vi "FTW-TestBootstrapper.vi"   [LabVIEW 2015, in "FTW-TestBootstrapper.lvclass"]
uses:
  FTW-TestBootstrapper.lvclass
panel:
  # "Static links to all FTW tests"
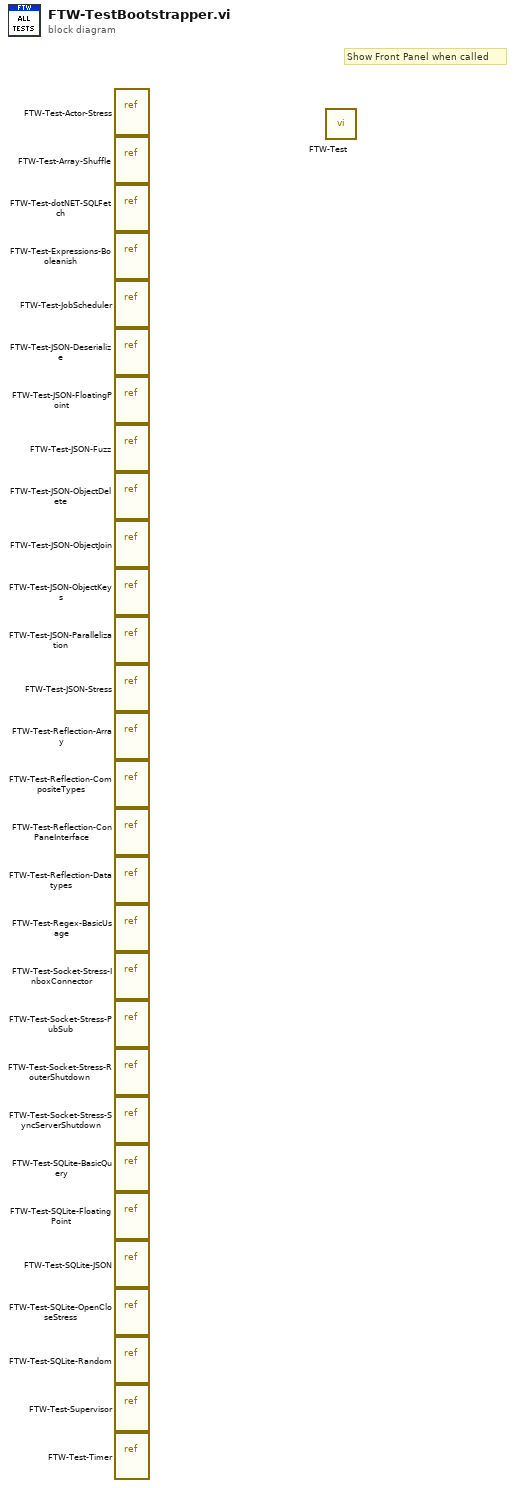
[diagram p0: block diagram]
diagram:
  # "Show Front Panel when called"
  n1 = vi-ref "FTW-Test-Actor-Stress.vi"() -> ()  [unwired: 1 out]
  n2 = vi-ref "FTW-Test-Array-Shuffle.vi"() -> ()  [unwired: 1 out]
  n3 = vi-ref "FTW-Test-dotNET-SQLFetch.vi"() -> ()  [unwired: 1 out]
  n4 = vi-ref "FTW-Test-Expressions-Booleanish.vi"() -> ()  [unwired: 1 out]
  n5 = vi-ref "FTW-Test-JobScheduler.vi"() -> ()  [unwired: 1 out]
  n6 = vi-ref "FTW-Test-JSON-Deserialize.vi"() -> ()  [unwired: 1 out]
  n7 = vi-ref "FTW-Test-JSON-FloatingPoint.vi"() -> ()  [unwired: 1 out]
  n8 = vi-ref "FTW-Test-JSON-Fuzz.vi"() -> ()  [unwired: 1 out]
  n9 = vi-ref "FTW-Test-JSON-ObjectDelete.vi"() -> ()  [unwired: 1 out]
  n10 = vi-ref "FTW-Test-JSON-ObjectJoin.vi"() -> ()  [unwired: 1 out]
  n11 = vi-ref "FTW-Test-JSON-ObjectKeys.vi"() -> ()  [unwired: 1 out]
  n12 = vi-ref "FTW-Test-JSON-Parallelization.vi"() -> ()  [unwired: 1 out]
  n13 = vi-ref "FTW-Test-JSON-Stress.vi"() -> ()  [unwired: 1 out]
  n14 = vi-ref "FTW-Test-Reflection-Array.vi"() -> ()  [unwired: 1 out]
  n15 = vi-ref "FTW-Test-Reflection-CompositeTypes.vi"() -> ()  [unwired: 1 out]
  n16 = vi-ref "FTW-Test-Reflection-ConPaneInterface.vi"() -> ()  [unwired: 1 out]
  n17 = vi-ref "FTW-Test-Reflection-Datatypes.vi"() -> ()  [unwired: 1 out]
  n18 = vi-ref "FTW-Test-Regex-BasicUsage.vi"() -> ()  [unwired: 1 out]
  n19 = vi-ref "FTW-Test-Socket-Stress-InboxConnector.vi"() -> ()  [unwired: 1 out]
  n20 = vi-ref "FTW-Test-Socket-Stress-PubSub.vi"() -> ()  [unwired: 1 out]
  n21 = vi-ref "FTW-Test-Socket-Stress-RouterShutdown.vi"() -> ()  [unwired: 1 out]
  n22 = vi-ref "FTW-Test-Socket-Stress-SyncServerShutdown.vi"() -> ()  [unwired: 1 out]
  n23 = vi-ref "FTW-Test-SQLite-BasicQuery.vi"() -> ()  [unwired: 1 out]
  n24 = vi-ref "FTW-Test-SQLite-FloatingPoint.vi"() -> ()  [unwired: 1 out]
  n25 = vi-ref "FTW-Test-SQLite-JSON.vi"() -> ()  [unwired: 1 out]
  n26 = vi-ref "FTW-Test-SQLite-OpenCloseStress.vi"() -> ()  [unwired: 1 out]
  n27 = vi-ref "FTW-Test-SQLite-Random.vi"() -> ()  [unwired: 1 out]
  n28 = vi-ref "FTW-Test-Supervisor.vi"() -> ()  [unwired: 1 out]
  n29 = vi-ref "FTW-Test-Timer.vi"() -> ()  [unwired: 1 out]
  n30 = call "FTW-Test.vi"() -> ()  [unwired: 12 in]
